vi "SerializeFaceEncoding.vi"(8 "error in (no error)":errorcluster, 11 "FaceEncoding in":refnum<k24>) -> (0 "error out":errorcluster, 2 "BinaryEncoding":u8[](array[numeric]), 3 "FaceEncoding Out":refnum<k24>)   [LabVIEW 2020, in "FaceRecognitionDotNet.lvlib" / "FaceRecognition.lvclass"]
uses:
  FaceRecognition.lvclass
  dll/FaceRecognitionDotNet.dll
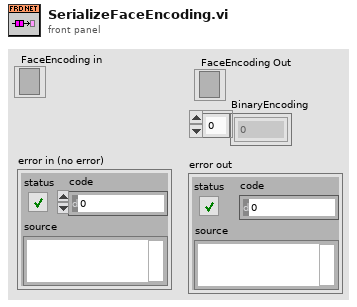
[diagram p1: front panel]
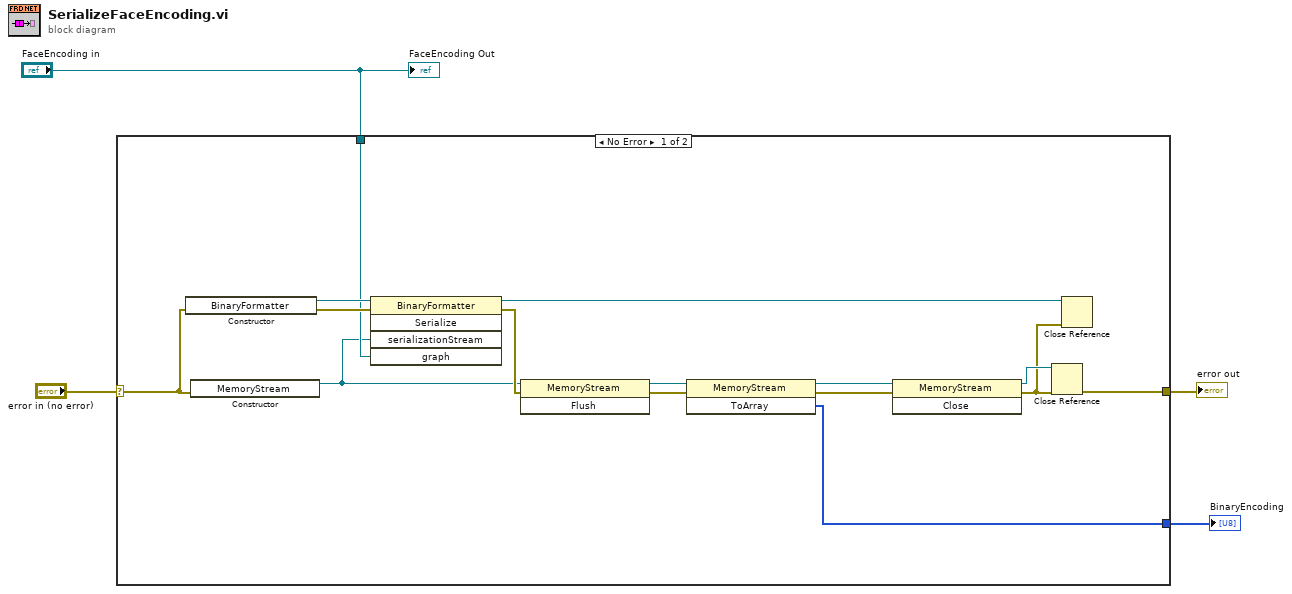
[diagram p0: block diagram]
diagram:
  n1 = case shown="No Error" "error in (no error)" {
    selector: "error in (no error)" -> [w8 w20]
    tunnel: "FaceEncoding in" -> [w12 _]
    tunnel: [w7 w20] -> w2
    tunnel: [w5 _] -> w1
    frame No Error {
      n2 = constructor class="BinaryFormatter"(error in=w8) -> (reference out=w15:refnum<k24>, error out=w16:errorcluster)  [unwired: 2 in, 1 out]
      n3 = constructor class="MemoryStream"(error in=w8) -> (reference out=w11:refnum<k24>)  [unwired: 2 in, 2 out]
      n4 = invoke class="BinaryFormatter" method="Serialize"(reference=w15, error in=w16, "serializationStream"=w11, "graph"=w12) -> (reference out=w17:refnum<k24>, error out=w18:errorcluster)  [unwired: 1 in, 3 out]
      n5 = invoke class="MemoryStream" method="Flush"(reference=w11, error in=w18) -> (reference out=w10:refnum<k24>, error out=w9:errorcluster)  [unwired: 1 in, 1 out]
      n6 = invoke class="MemoryStream" method="ToArray"(reference=w10, error in=w9) -> (reference out=w13:refnum<k24>, error out=w14:errorcluster, "ToArray"=w5:u8[])  [unwired: 1 in]
      n7 = invoke class="MemoryStream" method="Close"(reference=w13, error in=w14) -> (reference out=w19:refnum<k24>, error out=w6:errorcluster)  [unwired: 1 in, 1 out]
      n8 = Close Reference(reference=w19, error in (no error)=w6) -> (error out=w7:errorcluster)
      n9 = Close Reference(reference=w17, error in (no error)=w6) -> ()  [unwired: 1 out]
    }
    frame Error {
    }
  }
  "error out" <- w2
  "BinaryEncoding" <- w1
  "FaceEncoding Out" <- "FaceEncoding in"
